vi "Result.Overall Test Status to String.vi"(9 "Result State Str In":string, 10 "ResultState.State":T1) -> (1 "ResultState.State Out":T1, 2 "Result State Str":string)   [LabVIEW 2019]
uses:
  <vilib>/KATE/SeqMgr/SeqMgr.Result State Enum.ctl
  <vilib>/KATE/SeqMgr/SeqMgr.lvlib
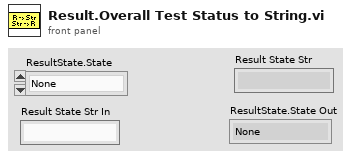
[diagram p1: front panel]
types:
  T1 = typedef "KATE_Lib.lvlib/SeqMgr.lvlib/SeqMgr.Result State Enum.ctl" = enum16{"None", "Passing", "Failing", "PASS", "FAIL", "ABORT", "ERROR"}
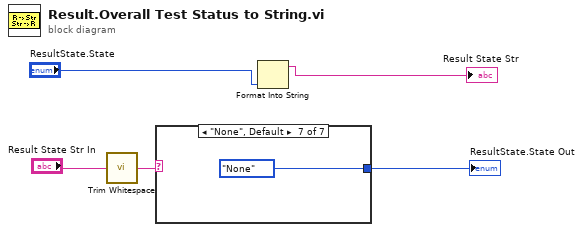
[diagram p0: block diagram]
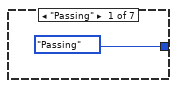
[diagram p2: hidden frame]
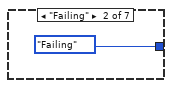
[diagram p3: hidden frame]
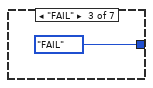
[diagram p4: hidden frame]
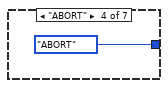
[diagram p5: hidden frame]
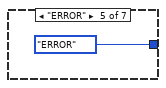
[diagram p6: hidden frame]
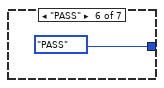
[diagram p7: hidden frame]
diagram:
  n1 = call <vilib>:"Trim Whitespace.vi"("string"="Result State Str In") -> ("trimmed string"=w2:string)  [unwired: 1 in]
  n2 = case shown="\"None\", Default" w2 {
    tunnel: [SeqMgr.Result_State_Enum."Passing" ("ResultState.State") SeqMgr.Result_State_Enum."Failing" ("ResultState.State") SeqMgr.Result_State_Enum."FAIL" ("ResultState.State") SeqMgr.Result_State_Enum."ABORT" ("ResultState.State") SeqMgr.Result_State_Enum."ERROR" ("ResultState.State") SeqMgr.Result_State_Enum."PASS" ("ResultState.State") SeqMgr.Result_State_Enum."None" ("ResultState.State")] -> w3
    frame "Passing" {
    }
    frame "Failing" {
    }
    frame "FAIL" {
    }
    frame "ABORT" {
    }
    frame "ERROR" {
    }
    frame "PASS" {
    }
    frame "None", Default {
    }
  }
  "ResultState.State Out" <- w3
  n3 = Format Into String("ResultState.State") -> (resulting string=→"Result State Str":string)  [unwired: 3 in, 1 out]
